vi "To and From Array Test.vi"() -> (0 "error out":errorcluster, 1 "Pass":bool, 2 "Lines Equal":bool, 3 "Class Equal":bool)   [LabVIEW 2014, in "io plugin tests.lvlib"]
uses:
  io plugin tests.lvlib
  module/configuration/tag bus configurable plugin module configuration.lvclass/tag bus configurable plugin module configuration.ctl
  <vilib>/NI/Tag Bus Module Framework/channel/TBM channel.lvclass
  module/configuration/tag bus configurable plugin module configuration.lvclass
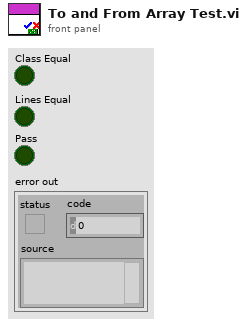
[diagram p1: front panel]
types:
  T1 = typedef "tag bus configurable plugin module configuration.lvclass/Line.ctl" = cluster{"channel":refnum<class "TBM channel.lvclass">}
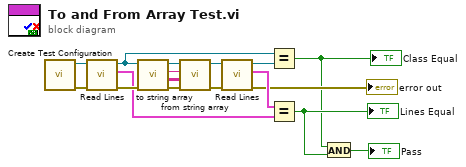
[diagram p0: block diagram]
diagram:
  n1 = call "Create Test Configuration.vi"() -> ("error out"=w9:errorcluster, "Module Configuration"=w10:refnum<class "tag bus configurable plugin module configuration.lvclass">)  [unwired: 6 in, 4 out]
  n2 = call "Read Lines.vi"("error in (no error)"=w9, "tag bus configurable plugin module configuration in"=w10) -> ("error out"=w11:errorcluster, "Lines"=w5:T1[], "tag bus configurable plugin module configuration out"=w7:refnum<class "tag bus configurable plugin module configuration.lvclass">)  [unwired: 7 in]
  n3 = call-dynamic "to string array.vi"("error in (no error)"=w11, "module configuration in"=w7) -> ("error out"=w17:errorcluster, "Array"=w16:string[][], "version"=w15:string, "module configuration out"=w14:refnum<class "tag bus configurable plugin module configuration.lvclass">)  [unwired: 6 in]
  n4 = call-dynamic "from string array.vi"("error in (no error)"=w17, "String Array"=w16, "version"=w15, "module configuration in"=w14) -> ("error out"=w12:errorcluster, "module configuration out"=w13:refnum<class "tag bus configurable plugin module configuration.lvclass">)  [unwired: 6 in]
  n5 = call "Read Lines.vi"("error in (no error)"=w12, "tag bus configurable plugin module configuration in"=w13) -> ("error out"=→"error out":errorcluster, "Lines"=w6:T1[], "tag bus configurable plugin module configuration out"=w8:refnum<class "tag bus configurable plugin module configuration.lvclass">)  [unwired: 7 in]
  n6 = Equal?(x=w7, y=w8) -> (x = y?=w1:bool)
  "Class Equal" <- w1
  n7 = Equal?(x=w6, y=w5) -> (x = y?=w2:bool)
  "Lines Equal" <- w2
  n8 = And(x=w1, y=w2) -> (x .and. y?=→"Pass":bool)
